vi "BuildStimulusPulse.vi"(1 "Phase shift angle":dbl, 6 "Sampling Rate (Hz)":dbl=10000.0, 7 "Pulse Type":enum16{"Monophasic", "Biphasic"}(ring), 8 "Num Pulses":u32=1 min=1, 9 "Inter-Pulse Interval (ms)":dbl=10.0, 10 "Pulse Width (ms)":dbl=0.5, 11 "Amplitude (Volts)":dbl=1.0) -> (0 "error out":errorcluster, 3 "Waveform Out":waveform(dbl), 4 "Final Array Size":i32)   [LabVIEW 2017]
panel:
  out "Pulse period":dbl
  out "Array":dbl[](array[numeric])
  out "Waveform Debug":waveform(dbl)(graph)
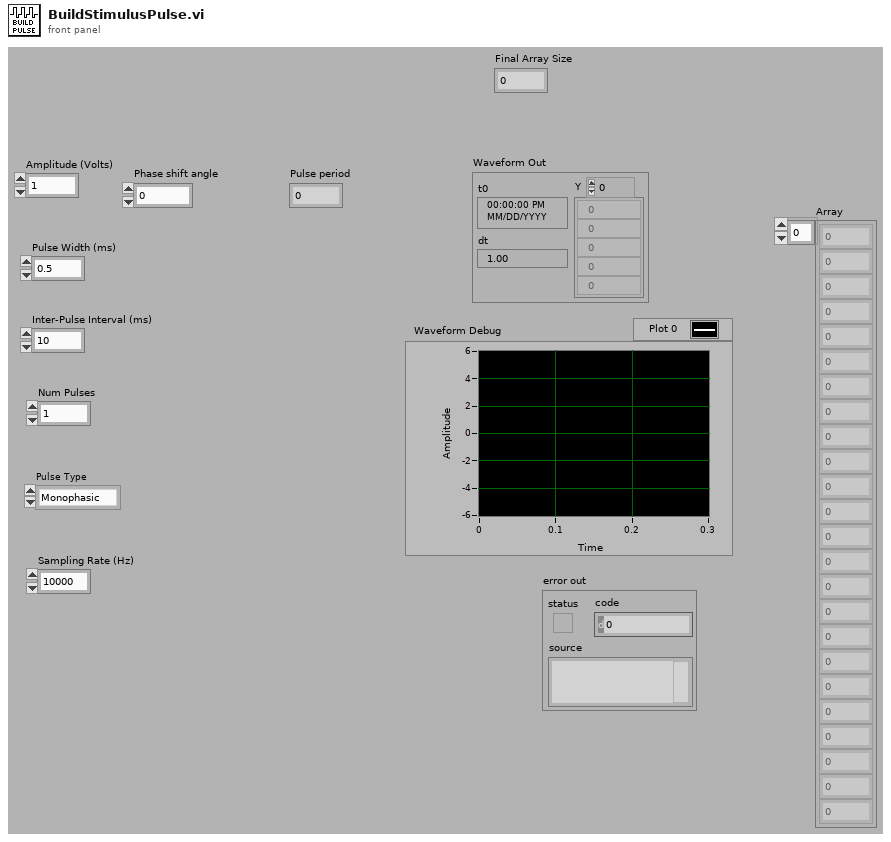
[diagram p1: front panel]
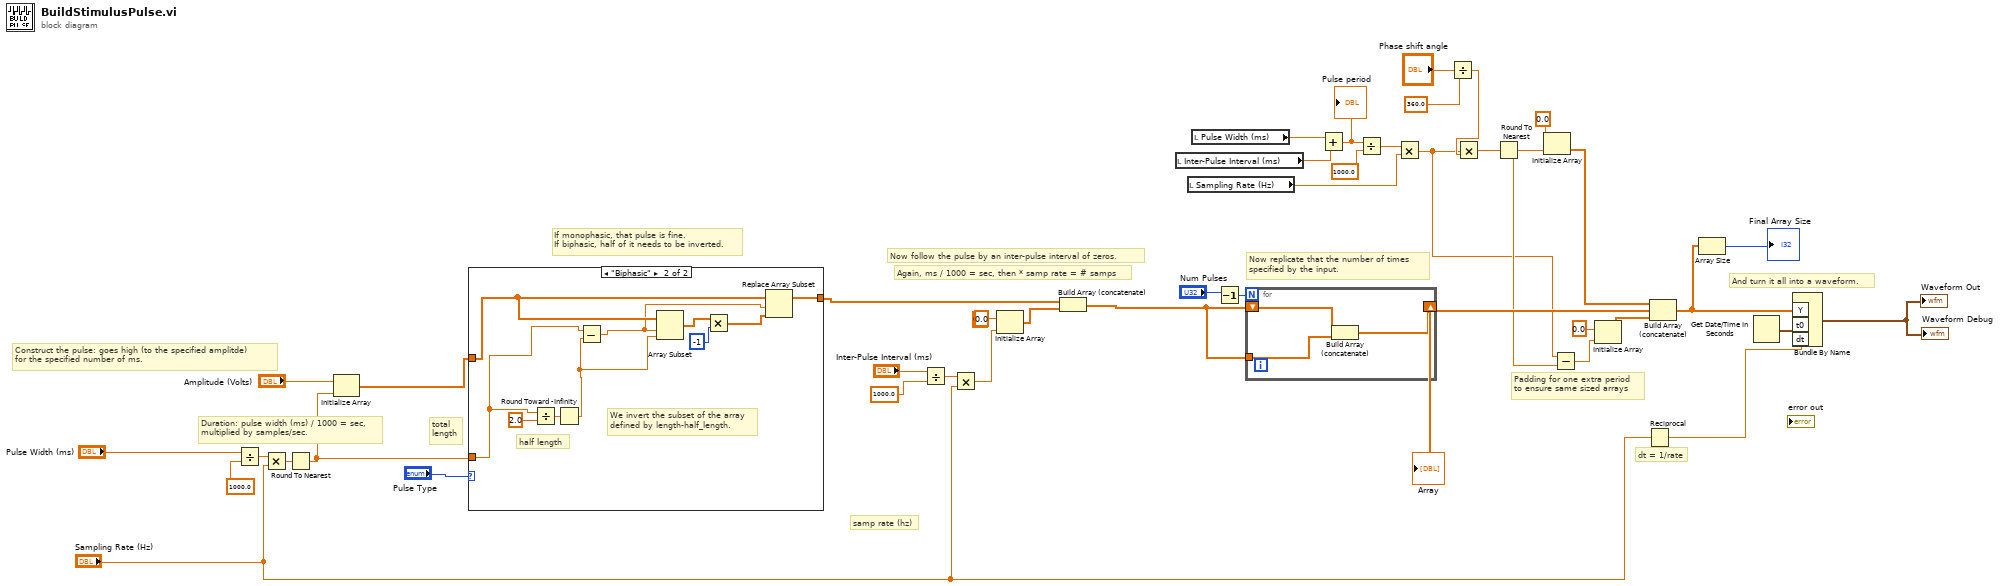
[diagram p0: block diagram]
diagram:
  (unwired) 0.0 ("element")
  # "Padding for one extra period\nto ensure same sized arrays"
  # "dt = 1/rate"
  # "And turn it all into a waveform."
  # "Now replicate that the number of times\nspecified by the input."
  # "samp rate (hz)"
  # "Again, ms / 1000 = sec, then * samp rate = # samps"
  # "total\nlength"
  # "Now follow the pulse by an inter-pulse interval of zeros."
  # "If monophasic, that pulse is fine.\nIf biphasic, half of it needs to be inverted."
  # "Duration: pulse width (ms) / 1000 = sec,\nmultiplied by samples/sec."
  # "Construct the pulse: goes high (to the specified amplitde)\nfor the specified number of ms."
  n1 = Divide(x="Pulse Width (ms)", y=1000.0) -> (x/y=w40:dbl)
  n2 = Multiply(x=w40, y="Sampling Rate (Hz)") -> (x*y=w39:dbl)
  n3 = Round To Nearest(number=w39) -> (nearest integer value=w37:dbl)
  n4 = Initialize Array("Amplitude (Volts)", w37) -> (w19:dbl[])
  n5 = case shown="\"Biphasic\"" "Pulse Type" {
    tunnel: w19 -> [w43 w51]
    tunnel: [w43 w45] -> w36
    tunnel: w37 -> [_ w44]
    frame "Monophasic", Default {
    }
    frame "Biphasic" {
      # "half length"
      # "We invert the subset of the array\ndefined by length-half_length."
      n6 = Divide(x=w44, y=2.0) -> (x/y=w49:dbl)
      n7 = Round Toward -Infinity(1:w49) -> (0:w48:dbl)
      n8 = Subtract(x=w44, y=w48) -> (x-y=w46:dbl)
      n9 = Array Subset(array=w51, index=w46, length=w48) -> (w52:dbl[])
      n10 = Multiply(x=w52, y=-1 ("Amplitude (Volts)")) -> (x*y=w47:dbl[])
      n11 = Replace Array Subset(array=w51, new element=w47, index=w46) -> (w45:dbl[])
    }
  }
  n12 = Divide(x="Inter-Pulse Interval (ms)", y=1000.0) -> (x/y=w33:dbl)
  n13 = Multiply(x=w33, y="Sampling Rate (Hz)") -> (x*y=w32:dbl)
  n14 = Initialize Array(0.0 ("element"), w32) -> (w35:dbl[])
  n15 = Build Array (concatenate)(w36, w35) -> (w28:dbl[])
  n16 = local read "Inter-Pulse Interval (ms)"() -> (w10:dbl)
  n17 = local read "Sampling Rate (Hz)"() -> (w6:dbl)
  n18 = local read "Pulse Width (ms)"() -> (w9:dbl)
  n19 = Decrement(x="Num Pulses") -> (x-1=w30:u32)
  n20 = for {
    N: w30 -> [_]
    shift-right: [w55] -> w21
    shift-left: w28 -> [w56]
    tunnel: w28 -> [w54]
    n21 = Build Array (concatenate)(w56, w54) -> (w55:dbl[])
  }
  "Array" <- w21
  n22 = Add(x=w9, y=w10) -> (x+y=w25:dbl)
  "Pulse period" <- w25
  n23 = Divide(x=w25, y=1000.0) -> (x/y=w12:dbl)
  n24 = Multiply(x=w12, y=w6) -> (x*y=w11:dbl)
  n25 = Divide(x="Phase shift angle", y=360.0) -> (x/y=w17:dbl)
  n26 = Multiply(x=w11, y=w17) -> (x*y=w24:dbl)
  n27 = Round To Nearest(number=w24) -> (nearest integer value=w14:dbl)
  n28 = Initialize Array(0.0 ("element"), w14) -> (w4:dbl[])
  n29 = Subtract(x=w11, y=w14) -> (x-y=w13:dbl)
  n30 = Initialize Array(0.0 ("element"), w13) -> (w16:dbl[])
  n31 = Reciprocal(x="Sampling Rate (Hz)") -> (1/x=w3:dbl)
  n32 = Build Array (concatenate)(w4, w21, w16) -> (w2:dbl[])
  n33 = Array Size(array=w2) -> (size(s)=→"Final Array Size":i32)
  n34 = Get Date/Time In Seconds() -> (seconds since 1Jan1904=w27:timestamp)
  n35 = Bundle By Name("Y"=w2, "t0"=w27, "dt"=w3) -> (→"Waveform Out" →"Waveform Debug":waveform(dbl))  [unwired: 1 in]
